vi "Test Configuration File Creates Non Existing File.vi"(8 "error in (no error)":errorcluster, 11 "Process Test In":refnum<class "Configuration File Process Interface Test.lvclass">) -> (0 "error out":errorcluster, 3 "Process Test Out":refnum<class "Configuration File Process Interface Test.lvclass">)   [LabVIEW 2020, in "Configuration File Process Interface Test.lvclass"]
uses:
  Configuration File Process Interface Test.lvclass
  C:/Program Files (x86)/National Instruments/LabVIEW 2020/vi.lib/Astemes/LUnit/Test Case.lvclass
  Mock Configurable Process/Mock Configurable Process.lvclass
  <vilib>/Astemes/LUnit/Test Case.lvclass/Test Case.ctl
  <vilib>/Astemes/LUnit/LUnit Assertion Result.lvclass/LUnit Assertion Result.ctl
  <vilib>/Astemes/LUnit/LUnit Test Case Result.lvclass/LUnit Test Case Result.ctl
  <vilib>/Astemes/LUnit/LUnit Method Result.lvclass/LUnit Method Result.ctl
  <vilib>/Astemes/LUnit/Palette/Fail.vi
  <vilib>/Astemes/LUnit/Palette/Pass.vi
  <vilib>/Astemes/LUnit/Set Assertion Type.vi
  <vilib>/Astemes/LUnit/Add test result.vi
  <vilib>/Astemes/LUnit/LUnit Write Passed.vi
  <vilib>/Astemes/LUnit/LUnit Write Message.vi
  <vilib>/Astemes/LUnit/LUnit Write Description.vi
  <vilib>/Astemes/LUnit/LUnit Write Assertion Type.vi
  <vilib>/Astemes/LUnit/LUnit Record Assertion Result.vi
  <vilib>/Astemes/LUnit/LUnit Aggregate Assertion Results.vi
  <vilib>/Astemes/LUnit/Assertion Result/LUnit Read Status.vi
  <vilib>/Astemes/LUnit/LUnit Read Message.vi
  <vilib>/Astemes/LUnit/LUnit Read Description.vi
  <vilib>/Astemes/LUnit/Method Result/LUnit Merge Status.vi
  <vilib>/Astemes/LUnit/LUnit Concatenate result strings.vi
  <vilib>/Astemes/LUnit/LUnit Assertion Result.lvclass
  Configuration File Process Interface Test.lvclass/Configuration File Process Interface Test.ctl
  <vilib>/Astemes/LUnit/Test Case.lvclass
  C:/Users/anton/Documents/GitHub/Triarc-Framework/source/Framework Test/Configuration Interface Test/Configuration Interface Test.lvclass
  C:/Users/anton/Documents/GitHub/Triarc-Framework/source/Framework Test/Configuration File Process Interface Test/Configuration File Process Interface Test.lvclass
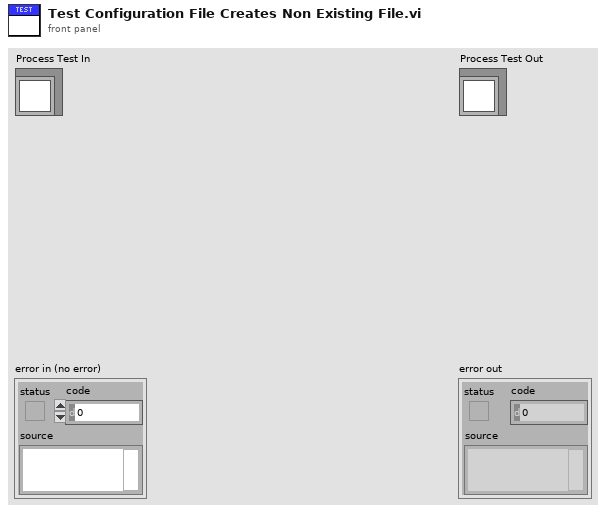
[diagram p1: front panel]
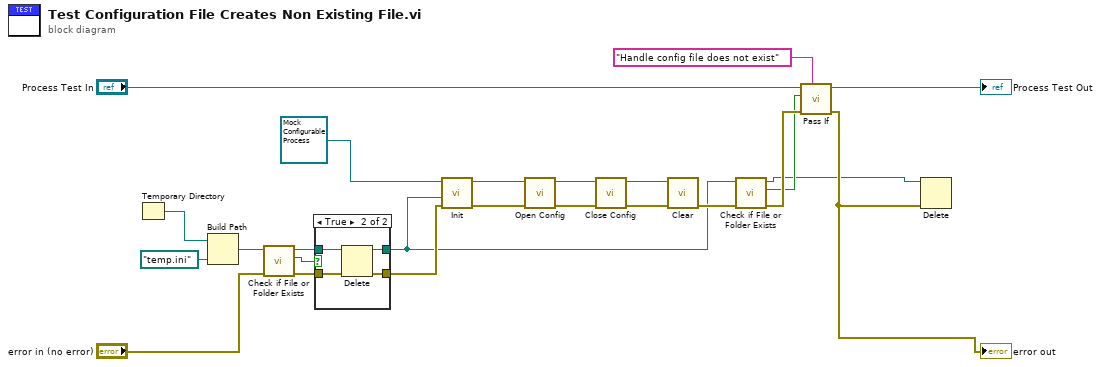
[diagram p0: block diagram]
diagram:
  n1 = Temporary Directory() -> (w19:path)
  n2 = Build Path(base path=w19, name or relative path=path "temp.ini") -> (appended path=w17:path)
  n3 = call <vilib>:"Check if File or Folder Exists.vi"("error in (no error)"="error in (no error)", "path"=w17) -> ("error out"=w12:errorcluster, "file or folder exists?"=w9:bool, "dup path"=w13:path)  [unwired: 7 in]
  n4 = case shown="True" w9 {
    tunnel: w13 -> [w26 w30]
    tunnel: [w26 w29] -> w6
    tunnel: w12 -> [w25 w28]
    tunnel: [w25 w27] -> w10
    frame False {
    }
    frame True {
      n5 = Delete(path (use dialog)=w30, error in=w28) -> (deleted path=w29:path, error out=w27:errorcluster)  [unwired: 3 in, 1 out]
    }
  }
  n6 = call-dynamic "Init.vi"("error in (no error)"=w10, "Config File Path"=w6, "Process In"=refnum<class "Mock Configurable Process.lvclass"> refnum ("Mock Configurable.lvclass")) -> ("error out"=w22:errorcluster, "Process Out"=w23:refnum<class "Mock Configurable Process.lvclass">)  [unwired: 7 in]
  n7 = call-dynamic "Open Config.vi"("error in (no error)"=w22, "Configuration File File In"=w23) -> ("error out"=w8:errorcluster, "Configuration File File Out"=w2:refnum<class "Mock Configurable Process.lvclass">)  [unwired: 8 in]
  n8 = call-dynamic "Close Config.vi"("error in (no error)"=w8, "Configuration File File In"=w2) -> ("error out"=w3:errorcluster, "Configuration File File Out"=w1:refnum<class "Mock Configurable Process.lvclass">)  [unwired: 8 in]
  n9 = call-dynamic "Clear.vi"("error in (no error)"=w3, "Process In"=w1) -> ("error out"=w16:errorcluster)  [unwired: 9 in]
  n10 = call <vilib>:"Check if File or Folder Exists.vi"("error in (no error)"=w16, "path"=w6) -> ("error out"=w15:errorcluster, "file or folder exists?"=w14:bool, "dup path"=w5:path)  [unwired: 7 in]
  n11 = call <vilib>:"Pass If.vi"("Description"="Handle config file does not exist", "error in (no error)"=w15, "Pass?"=w14, "LUnit Test Case In"="Process Test In") -> ("error out"=w7:errorcluster, "LUnit Test Case Out"=→"Process Test Out":refnum<class "Configuration File Process Interface Test.lvclass">)  [unwired: 6 in]
  "error out" <- w7
  n12 = Delete(path (use dialog)=w5, error in=w7) -> ()  [unwired: 3 in, 3 out]
